vi "Add Pending Response.vi"(8 "Error In":errorcluster, 10 "Expected Response":refnum<class "CANopen Response Message.lvclass">, 11 "reference in":refnum<class "SDO Manager.lvclass">) -> (0 "Error Out":errorcluster, 1 "Response Notifier out":refnum<notifier>, 3 "reference out":refnum<class "SDO Manager.lvclass">)   [LabVIEW 2024, in "CANopen Master.lvlib" / "SDO Manager.lvclass"]
uses:
  SDO Manager.lvclass
  CANopen Response/CANopen Response Message.lvclass
  CANopen Message/CANopen Message.lvclass
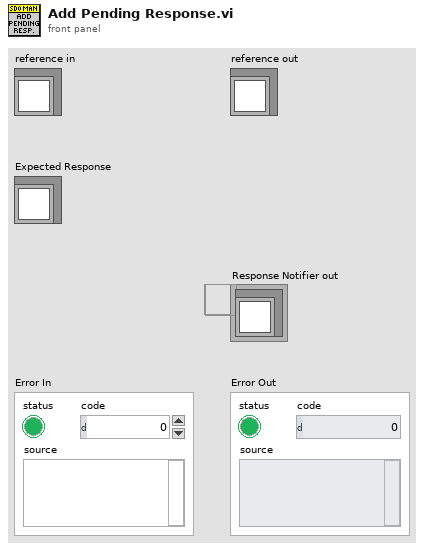
[diagram p1: front panel]
types:
  T1 = typedef "CANopen Master.lvlib/SDO Manager.lvclass/ObjectAttributes.ctl" = cluster{"SDO Response Map":map{u32, refnum<notifier>}}
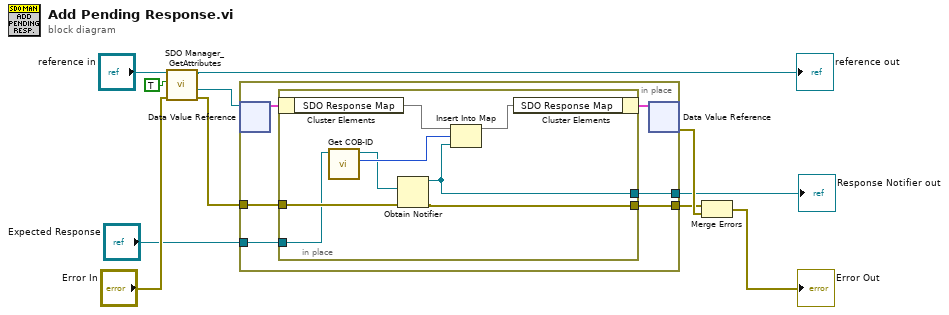
[diagram p0: block diagram]
diagram:
  n1 = call "SDO Manager_GetAttributes.vi"("Error In"="Error In", "OnlyGetDvrReference(False)"=TRUE, "reference in"="reference in") -> ("Error Out"=w8:errorcluster, "DataRef"=w11:refnum<data-value>, "reference out"=→"reference out":refnum<class "SDO Manager.lvclass">)  [unwired: 5 in, 1 out]
  n2 = in-place {
    in-place-border: [w17] -> w4
    in-place-border: w8 -> [w16]
    in-place-border: "Expected Response" -> [w15]
    in-place-border: [w14] -> w9
    n3 = in-place-dvr #1(w11) -> (w13:T1)  [unwired: 1 out]
    n4 = in-place {
      in-place-border: [w25] -> w17
      in-place-border: w16 -> [w23]
      in-place-border: w15 -> [w19]
      in-place-border: [w22] -> w14
      n5 = in-place-cluster #2(w13) -> ("SDO Response Map"=w21:map{u32, refnum<notifier>})
      n6 = call "Get COB-ID.vi"("CANopen Message in"=w19) -> ("COB-ID"=w24:u32, "CANopen Message out"=w18:refnum<class "CANopen Response Message.lvclass">)  [unwired: 9 in]
      n7 = Obtain Notifier(notification data type=w18, error in (no error)=w23) -> (notifier out=w25:refnum<notifier>, error out=w22:errorcluster)  [unwired: 2 in, 1 out]
      n8 = Insert Into Map(map in=w21, key=w24, value=w25) -> (map out=w20:map{u32, refnum<notifier>})  [unwired: 2 out]
      n9 = in-place-cluster #2("SDO Response Map"=w20) -> (w12:T1)
    }
    n10 = in-place-dvr #1(w12) -> (w10:errorcluster)  [unwired: 1 out]
  }
  "Response Notifier out" <- w4
  n11 = Merge Errors(w9, w10) -> (→"Error Out":errorcluster)
